vi "result file write header.vi"(8 "error in (no error)":errorcluster, 9 "measurement definition":T5, 10 "measdata definition":T1 {"Current Magnetic\nField\n(430 TCP reading)"."phi (deg)" format="%#_3g"}, 11 "refnum":refnum<file>) -> (0 "error out":errorcluster, 3 "refnum out":refnum<file>)   [LabVIEW 2013]
uses:
  measconfig cluster.ctl
  measurement sweep parameter.ctl
  devices/magnet/magnet polar field.ctl
  measdata cluster.ctl
  devices/magnet/AMI reading polar field.ctl
  devices/vna/vna data formats.ctl
  <vilib>/Utility/VariantDataType/VariantType.lvlib
panel:
  # "List of measurement data for the S-parameters."
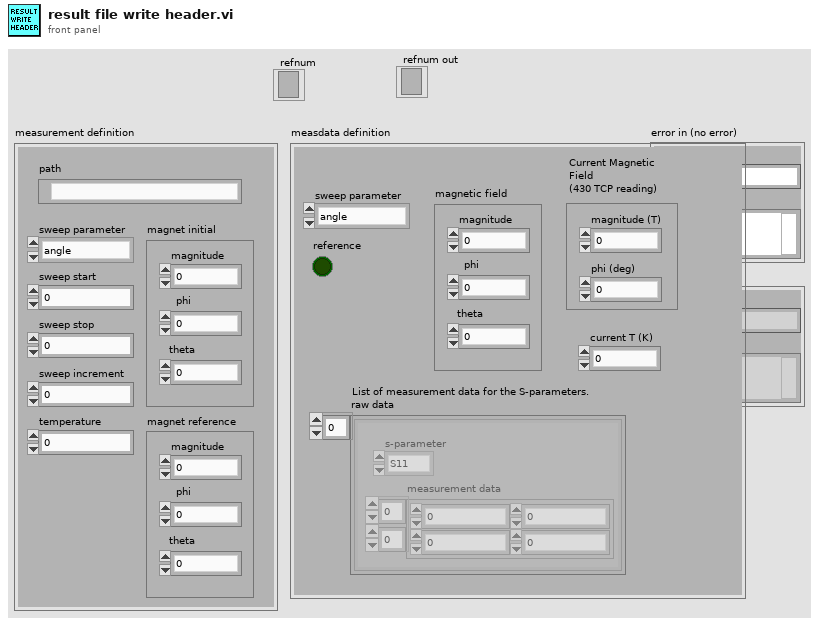
[diagram p1: front panel]
types:
  T1 = typedef "measdata cluster.ctl" = cluster{"raw data":cluster{"measurement data":dbl[][], "s-parameter":enum16{"S11", "S12", "S21", "S22"}}[], "magnetic field":T2, "reference":bool, "sweep parameter":T3, "Current Magnetic\nField\n(430 TCP reading)":T4, "current T (K)":dbl}
  T2 = typedef "magnet polar field.ctl" = cluster{"magnitude":dbl, "phi":dbl, "theta":dbl}
  T3 = typedef "measurement sweep parameter.ctl" = enum16{"angle", "magnetic field"}
  T4 = typedef "AMI reading polar field.ctl" = cluster{"magnitude (T)":dbl, "phi (deg)":dbl}
  T5 = typedef "measconfig cluster.ctl" = cluster{"sweep parameter":T3, "sweep start":dbl, "sweep stop":dbl, "sweep increment":dbl, "temperature":dbl, "path":path, "magnet initial":T2, "magnet reference":T2}
  T6 = typedef "vna data formats.ctl" = enum16{"FREQ", "MLIN", "MLOG", "PHAS", "REAL", "IMAG"}
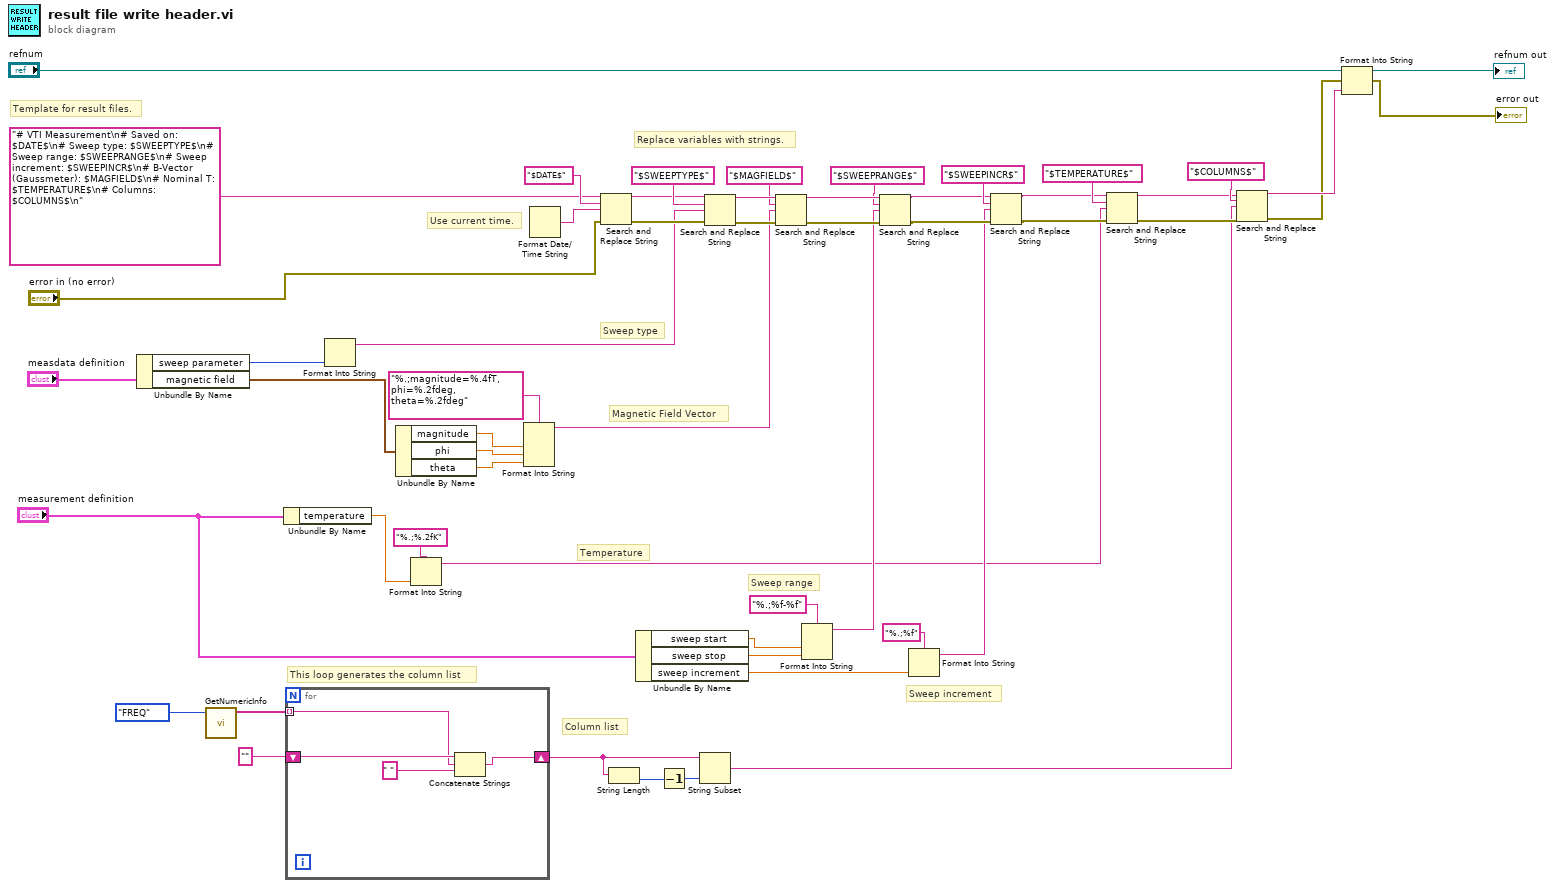
[diagram p0: block diagram]
diagram:
  # "Temperature"
  # "Replace variables with strings."
  # "Use current time."
  # "This loop generates the column list"
  # "Column list"
  # "Sweep increment"
  # "Sweep type"
  # "Magnetic Field Vector"
  # "Sweep range"
  # "Template for result files."
  n1 = Unbundle By Name("measdata definition") -> ("sweep parameter"=w8:T3, "magnetic field"=w6:T2)
  n2 = call <vilib>:"GetNumericInfo.vi"("Variant"=vna_data_formats."FREQ" ("data format")) -> ("EnumNames"=w19:string[])  [unwired: 7 in, 3 out]
  n3 = Unbundle By Name("measurement definition") -> ("temperature"=w18:dbl)
  n4 = for {
    shift-right: [w57] -> w2
    shift-left: "" -> [w58]
    tunnel: w19 -> [w56] mode=indexing
    n5 = Concatenate Strings(w58, w56, " ") -> (w57:string)
  }
  n6 = Format Into String(w8) -> (resulting string=w7:string)  [unwired: 3 in, 1 out]
  n7 = Unbundle By Name(w6) -> ("magnitude"=w11:dbl, "phi"=w10:dbl, "theta"=w9:dbl)
  n8 = Format Into String(format string="%.;%.2fK", w18) -> (resulting string=w15:string)  [unwired: 2 in, 1 out]
  n9 = Format Into String(format string="%.;magnitude=%.4fT, phi=%.2fdeg, theta=%.2fdeg", w11, w10, w9) -> (resulting string=w51:string)  [unwired: 2 in, 1 out]
  n10 = Format Date/Time String() -> (date/time string=w48:string)  [unwired: 3 in]
  n11 = Search and Replace String(input string="# VTI Measurement\n# Saved on: $DATE$\n# Sweep type: $SWEEPTYPE$\n# Sweep range: $SWEEPRANGE$\n# Sweep increment: $SWEEPINCR$\n# B-Vector (Gaussmeter): $MAGFIELD$\n# Nominal T: $TEMPERATURE$\n# Columns: $COLUMNS$\n", search string="$DATE$", replace string=w48, error in="error in (no error)") -> (result string=w46:string, error out=w49:errorcluster)  [unwired: 4 in, 2 out]
  n12 = String Length(string=w2) -> (length=w4:i32)
  n13 = Unbundle By Name("measurement definition") -> ("sweep start"=w41:dbl, "sweep stop"=w40:dbl, "sweep increment"=w38:dbl)
  n14 = Decrement(x=w4) -> (x-1=w3:i32)
  n15 = String Subset(string=w2, length (rest)=w3) -> (substring=w1:string)  [unwired: 1 in]
  n16 = Search and Replace String(input string=w46, search string="$SWEEPTYPE$", replace string=w7, error in=w49) -> (result string=w52:string, error out=w53:errorcluster)  [unwired: 4 in, 2 out]
  n17 = Search and Replace String(input string=w52, search string="$MAGFIELD$", replace string=w51, error in=w53) -> (result string=w44:string, error out=w43:errorcluster)  [unwired: 4 in, 2 out]
  n18 = Format Into String(format string="%.;%f-%f", w41, w40) -> (resulting string=w37:string)  [unwired: 2 in, 1 out]
  n19 = Search and Replace String(input string=w44, search string="$SWEEPRANGE$", replace string=w37, error in=w43) -> (result string=w33:string, error out=w34:errorcluster)  [unwired: 4 in, 2 out]
  n20 = Format Into String(format string="%.;%f", w38) -> (resulting string=w32:string)  [unwired: 2 in, 1 out]
  n21 = Search and Replace String(input string=w33, search string="$SWEEPINCR$", replace string=w32, error in=w34) -> (result string=w29:string, error out=w30:errorcluster)  [unwired: 4 in, 2 out]
  n22 = Search and Replace String(input string=w29, search string="$TEMPERATURE$", replace string=w15, error in=w30) -> (result string=w14:string, error out=w13:errorcluster)  [unwired: 4 in, 2 out]
  n23 = Search and Replace String(input string=w14, search string="$COLUMNS$", replace string=w1, error in=w13) -> (result string=w23:string, error out=w22:errorcluster)  [unwired: 4 in, 2 out]
  n24 = Format Into String(initial string="refnum", error in=w22, w23) -> (resulting string=→"refnum out":refnum<file>, error out=→"error out":errorcluster)  [unwired: 1 in]
